vi "AddItems.vi"(6 "Veg":bool, 7 "Price":i32, 8 "Error In":errorcluster, 9 "Description":string, 10 "Name":string, 11 "reference in":refnum<class "DinnerMenu.lvclass">) -> (0 "Error Out":errorcluster, 3 "reference out":refnum<class "DinnerMenu.lvclass">)   [LabVIEW 2020, in "DinnerMenu.lvclass"]
uses:
  DinnerMenu.lvclass
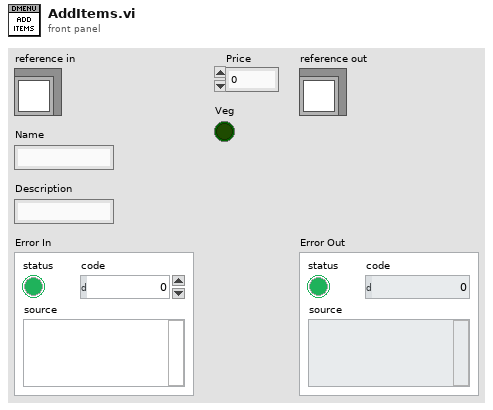
[diagram p1: front panel]
types:
  T1 = typedef "DinnerMenu.lvclass/ObjectAttributes.ctl" = cluster{"Max":i32, "_count":i32, "_items":refnum<class "Menu.lvclass">[], "Items":refnum<class "IEnumerable.lvclass">}
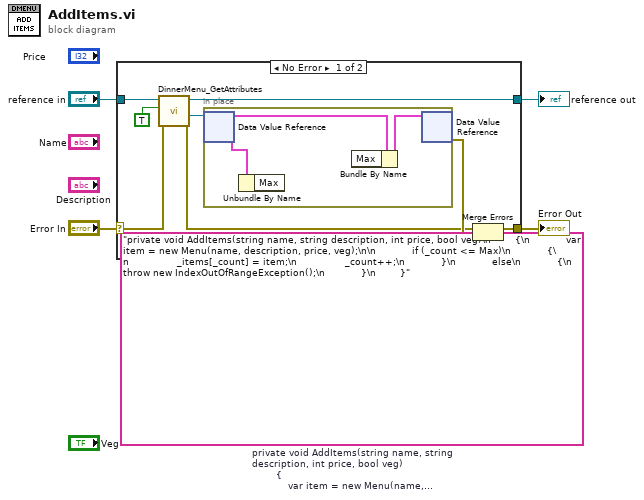
[diagram p0: block diagram]
diagram:
  (unwired) "private void AddItems(string name, string description, int price, bool veg)\n        {\n            var item = new Menu(name, description, price, veg);\n\n            if (_count <= Max)\n            {\n                _items[_count] = item;\n                _count++;\n            }\n            else\n            {\n                throw new IndexOutOfRangeException();\n            }\n        }"  # private void AddItems(string name, string description, int price, bool veg)         {             var item = new Menu(name, description, price, veg);              if (_count <= Max)             {                 _items[_count] = item;                 _count++;             }             else             {                 throw new IndexOutOfRangeException();             }         }
  n1 = case shown="No Error" "Error In" {
    selector: "Error In" -> [w11 w16]
    tunnel: [w8 w16] -> w3
    tunnel: [w9 w15] -> w1
    tunnel: "reference in" -> [w12 w15]
    frame No Error {
      n2 = call "DinnerMenu_GetAttributes.vi"("error in (no error)"=w11, "OnlyGetDvrReference(False)"=TRUE, "reference in"=w12) -> ("error out"=w6:errorcluster, "DataRef"=w7:refnum<data-value>, "reference out"=w9:refnum<class "DinnerMenu.lvclass">)  [unwired: 5 in, 1 out]
      n3 = in-place {
        n4 = in-place-dvr #1(w7) -> (w13:T1)  [unwired: 1 out]
        n5 = Unbundle By Name(w13) -> ()  [unwired: 1 out]
        n6 = Bundle By Name(cluster=w13) -> (w14:T1)  [unwired: 1 in]
        n7 = in-place-dvr #1(w14) -> (w10:errorcluster)  [unwired: 1 out]
      }
      n8 = Merge Errors(w6, w10) -> (w8:errorcluster)
    }
    frame Error {
    }
  }
  "Error Out" <- w3
  "reference out" <- w1
